vi "Configure Integration.vi"(8 "error in (no error)":errorcluster, 9 "Integration Time (1 PLCs)":dbl(ring)=1.0 items=["0.001"=0.001, "0.002"=0.002, "0.006"=0.006, "0.02"=0.02, "0.06"=0.06, "0.2"=0.2, "1"=1.0, "10"=10.0, "100"=100.0], 10 "Function (0: DC Voltage)":u16(ring) items=["DC Voltage", "AC Voltage", "2 - Wire Resistance", "4 - Wire Resistance", "DC Current", "AC Current", "Frequency", "Period", "Continuity", "Diode Checking", "VDC:VDC Ratio", "Temperature", "Capacitance"], 11 "VISA resource name":refnum<visa-resource-name>) -> (0 "error out":errorcluster, 3 "VISA resource name out":refnum<visa-resource-name>)   [LabVIEW 2013, in "Agilent 34401.lvlib"]
doc: "Configures the amount of time the analog to digital converter samples a signal. A longer integration time leads to a higher resolution. Auto Ranging must be disabled for these settings to apply.\n\n<b>Applicable Functions:</b>\n\nAll models:\n DC Voltage\n 2-Wire Resistance\n 4-Wire Resistance\n DC Current\n34401 only:\n DC Voltage Ratio\n34410/34411 only:\n Temperature\n\n<B>Note:</B>\n\nChanging the integration time may change the resolution configured in the <B>Configure Measurement VI</B>."
uses:
  <instrlib>/Agilent 34401/Agilent 34401.lvlib
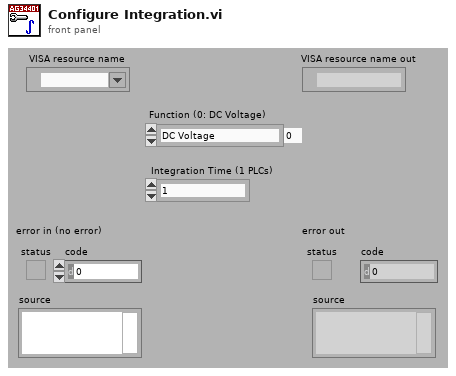
[diagram p1: front panel]
types:
  T1 = typedef "Agilent 34401.lvlib/Extended User Data.ctl" = cluster{"Trigger Source":u16, "Math Storage":u16, "Agilent Model":i32}
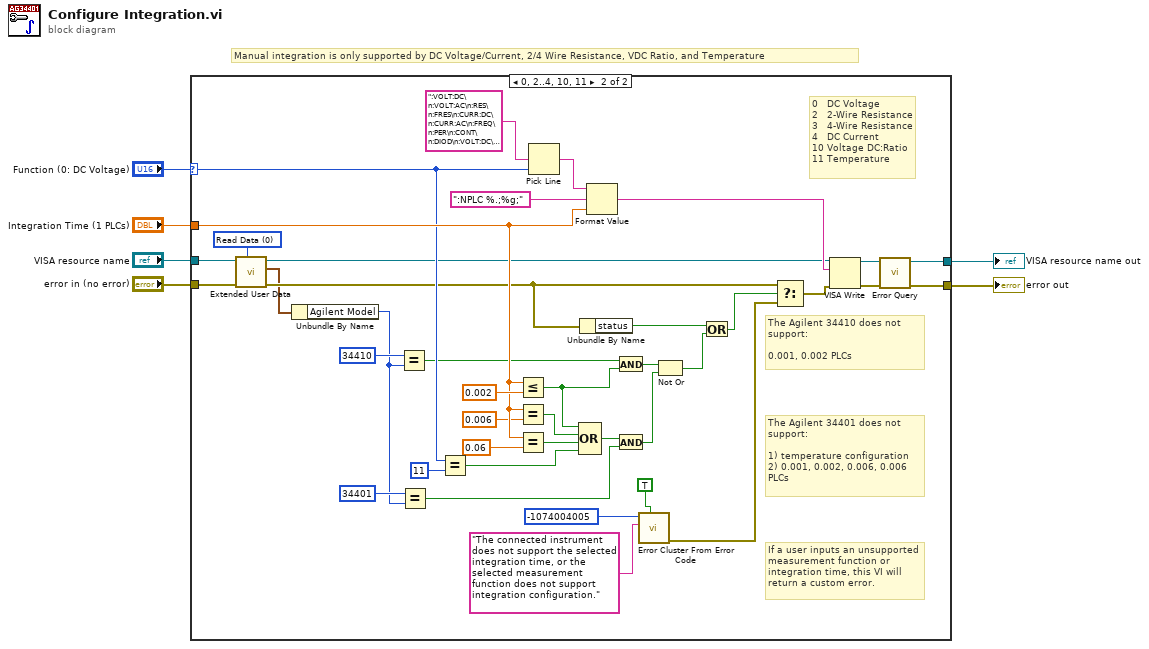
[diagram p0: block diagram]
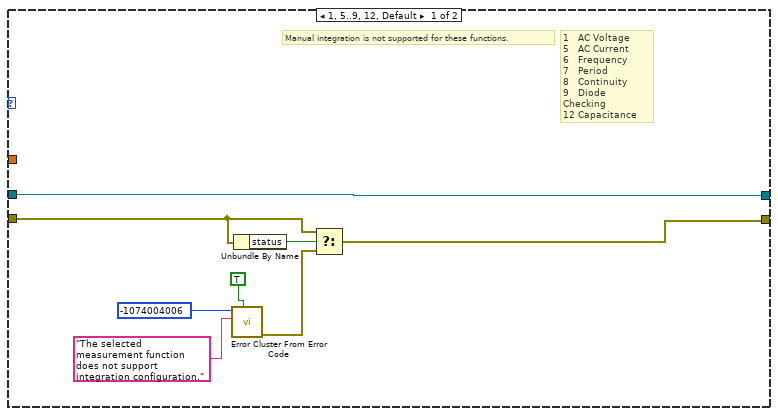
[diagram p2: hidden frame]
diagram:
  # "Manual integration is only supported by DC Voltage/Current, 2/4 Wire Resistance, VDC Ratio, and Temperature"
  n1 = case shown="0, 2..4, 10, 11" "Function (0: DC Voltage)" {
    selector: "Function (0: DC Voltage)" -> [_ w41]
    tunnel: "VISA resource name" -> [w14 w20]
    tunnel: "error in (no error)" -> [w9 w21]
    tunnel: [w14 w49] -> w3
    tunnel: [w7 w48] -> w2
    tunnel: "Integration Time (1 PLCs)" -> [_ w44]
    frame 1, 5..9, 12, Default {
      # "1   AC Voltage\n5   AC Current\n6   Frequency\n7   Period\n8   Continuity\n9   Diode Checking\n12 Capacitance"
      # "Manual integration is not supported for these functions."
      n2 = call <vilib>:"Error Cluster From Error Code.vi"("show call chain? (False)"=TRUE, "error message (\"\")"="The selected measurement function does not support integration configuration." ("Source (VI Name)"), "error code (0)"=-1074004006 ("Code")) -> ("error out"=w8:errorcluster)  [unwired: 6 in]
      n3 = Unbundle By Name(w9) -> ("status"=w10:bool)
      n4 = Select(t=w9, s=w10, f=w8) -> (s? t:f=w7:errorcluster)
    }
    frame 0, 2..4, 10, 11 {
      w17 = u16 0 items=["Read Data", "Write Data", "Dispose of Data"] ("Action")
      # "If a user inputs an unsupported measurement function or integration time, this VI will return a custom error."
      # "The Agilent 34401 does not support:\n\n1) temperature configuration\n2) 0.001, 0.002, 0.006, 0.006 PLCs"
      # "The Agilent 34410 does not support: \n\n0.001, 0.002 PLCs"
      # "0   DC Voltage\n2   2-Wire Resistance\n3   4-Wire Resistance\n4   DC Current\n10 Voltage DC:Ratio\n11 Temperature"
      n5 = call <instrlib>:"Extended User Data.vi"("Action"=w17, "Error In (no error)"=w21, "VISA resource name in"=w20) -> ("Error Out"=w19:errorcluster, "User Data Out"=w16:T1, "VISA resource name out"=w18:refnum<visa-resource-name>)  [unwired: 6 in]
      n6 = Unbundle By Name(w16) -> ("Agilent Model"=w15:i32)
      n7 = Equal?(x=34410, y=w15) -> (x = y?=w39:bool)
      n8 = Equal?(x=34401, y=w15) -> (x = y?=w35:bool)
      n9 = Equal?(x=w41, y=u16 11) -> (x = y?=w36:bool)
      n10 = Less Or Equal?(x=w44, y=0.002) -> (x <= y?=w31:bool)
      n11 = Equal?(x=w44, y=0.006) -> (x = y?=w38:bool)
      n12 = Equal?(x=w44, y=0.06) -> (x = y?=w37:bool)
      n13 = Pick Line(multi-line string=":VOLT:DC\n:VOLT:AC\n:RES\n:FRES\n:CURR:DC\n:CURR:AC\n:FREQ\n:PER\n:CONT\n:DIOD\n:VOLT:DC\n:TEMP\n:CAP", line index=w41) -> (output string=w50:string)  [unwired: 1 in]
      n14 = Compound Arithmetic op=OR(w31, w38, w37, w36) -> (w34:bool)
      n15 = Unbundle By Name(w19) -> ("status"=w23:bool)
      n16 = Format Value(string ("")=w50, format string=":NPLC %.;%g;", value (0)=w44) -> (output string=w27:string)
      n17 = And(x=w39, y=w31) -> (x .and. y?=w33:bool)
      n18 = And(x=w34, y=w35) -> (x .and. y?=w32:bool)
      n19 = call <vilib>:"Error Cluster From Error Code.vi"("show call chain? (False)"=TRUE, "error message (\"\")"="The connected instrument does not support the selected integration time, or the selected measurement function does not support integration configuration." ("Source (VI Name)"), "error code (0)"=-1074004005 ("Code")) -> ("error out"=w25:errorcluster)  [unwired: 6 in]
      n20 = Not Or(1:w32, 2:w33) -> (0:w24:bool)
      n21 = Or(x=w23, y=w24) -> (x .or. y?=w22:bool)
      n22 = Select(t=w19, s=w22, f=w25) -> (s? t:f=w26:errorcluster)
      n23 = VISA Write(VISA resource name=w18, write buffer=w27, error in (no error)=w26) -> (VISA resource name out=w53:refnum<visa-resource-name>, error out=w52:errorcluster)  [unwired: 1 out]
      n24 = call <instrlib>:"Error Query.vi"("error in (no error)"=w52, "VISA resource name"=w53) -> ("error out"=w48:errorcluster, "VISA resource name out"=w49:refnum<visa-resource-name>)  [unwired: 6 in, 2 out]
    }
  }
  "error out" <- w2
  "VISA resource name out" <- w3
